vi "Send Acknowledge Execution.vi"(7 "Priority":T1=enum."Normal" caption="Message Priority (Normal)", 8 "error in (no error)":errorcluster, 10 "VI Refnum":refnum<vi>, 11 "Message Enqueuer in":refnum<class "Message Enqueuer.lvclass">) -> (0 "error out":errorcluster, 3 "Message Enqueuer out":refnum<class "Message Enqueuer.lvclass">)   [LabVIEW 2021, in "Async Methods Actor.lvlib" / "Acknowledge Execution Msg.lvclass"]
doc: "Sends the <b>Async Methods Actor.lvlib:Acknowledge Execution Msg.lvclass</b> message.\n\nThis message will call <b>Acknowledge Execution.vi</b> on the <b>Async Methods Actor.lvlib:Async Methods Actor.lvclass</b> actor.\n\n<b>Acknowledge Execution.vi Description</b>"
uses:
  Acknowledge Execution Msg.lvclass
  Acknowledge Execution Msg.lvclass/Acknowledge Execution Msg.ctl
  <vilib>/ActorFramework/Message Enqueuer/Message Enqueuer.lvclass
  C:/Program Files/National Instruments/LabVIEW 2021/vi.lib/ActorFramework/Message/Message.lvclass
  C:/Projects/Async Methods Actor/Async Methods Actor/Async Methods Actor Messages/Acknowledge Execution Msg/Acknowledge Execution Msg.lvclass
  <vilib>/ActorFramework/Message Enqueuer/Message Priority.ctl
  <vilib>/ActorFramework/Actor/Actor.lvclass
  Async Message/Async Message.lvclass
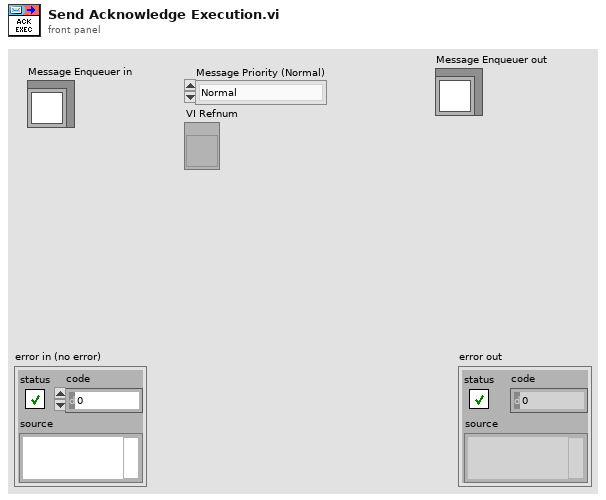
[diagram p1: front panel]
types:
  T1 = typedef "Actor Framework.lvlib/Message Enqueuer.lvclass/Message Priority.ctl" = enum16{"Low", "Normal", "High"}
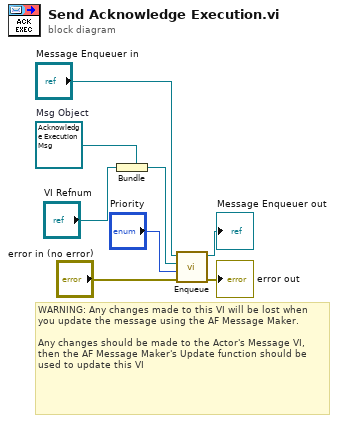
[diagram p0: block diagram]
diagram:
  w7 = refnum<class "Acknowledge Execution Msg.lvclass"> refnum  # Msg Object
  # "WARNING: Any changes made to this VI will be lost when you update the message using the AF Message Maker.\n\nAny changes should be made to the Actor's Message VI, then the AF Message Maker's Update function should be used to update this VI"
  n1 = Bundle(cluster=w7, "VI Refnum") -> (w2:refnum<class "Acknowledge Execution Msg.lvclass">)
  n2 = call <vilib>:"Enqueue.vi"("error in (no error)"="error in (no error)", "Message Priority (Normal)"="Priority", "Message"=w2, "Message Enqueuer in"="Message Enqueuer in") -> ("error out"=→"error out":errorcluster, "Message Enqueuer out"=→"Message Enqueuer out":refnum<class "Message Enqueuer.lvclass">)  [unwired: 6 in]
